vi "initial_feedback.vi"(1 "input cluster":T3) -> (0 "output cluster":T4)   [LabVIEW 2015]
uses:
  <vilib>/vision/Avi1.llb/AviRefnum.ctl
  <vilib>/userdefined/High Color/IMAQdx.ctl
  MWT.dll
panel:
  out "return type 2":i32
  out "return type":i32
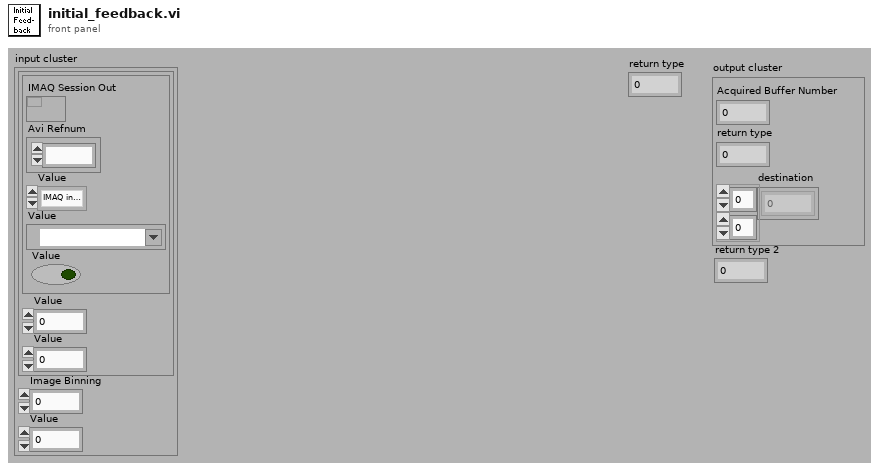
[diagram p1: front panel]
types:
  T1 = typedef "AviRefnum.ctl" = refnum<k1>
  T2 = typedef "IMAQdx.ctl" = refnum<k21>
  T3 = cluster{cluster{cluster{"IMAQ Session Out":refnum<k11>, "Avi Refnum":T1, "Value":enum32{"IMAQ interface", "IMAQdx interface", "AVI file"}, "Value":T2, "Value":bool}, "Value":i32, "Value":i32}, "Image Binning":u16, "Value":u16}
  T4 = cluster{"Acquired Buffer Number":i32, "return type":i32, "destination":i16[][]}
  T5 = typedef "Image Type" = u32
  T6 = typedef "IMAQ Image.ctl" = refnum<image>
  T7 = cluster{cluster{"IMAQ Session Out":refnum<k11>, "Avi Refnum":T1, "Value":enum32{"IMAQ interface", "IMAQdx interface", "AVI file"}, "Value":T2, "Value":bool}, "Value":i32, "Value":i32}
  T8 = cluster{"IMAQ Session Out":refnum<k11>, "Avi Refnum":T1, "Value":enum32{"IMAQ interface", "IMAQdx interface", "AVI file"}, "Value":T2, "Value":bool}
  T9 = cluster{cluster{"IMAQ Session Out":refnum<k11>, "Avi Refnum":T1, "Value":enum32{"IMAQ interface", "IMAQdx interface", "AVI file"}, "Value":T2, "Value":bool}, "Value":i32}
  T10 = cluster{"Acquired Buffer Number":i32, "return type":i32, "image":i16[][]}
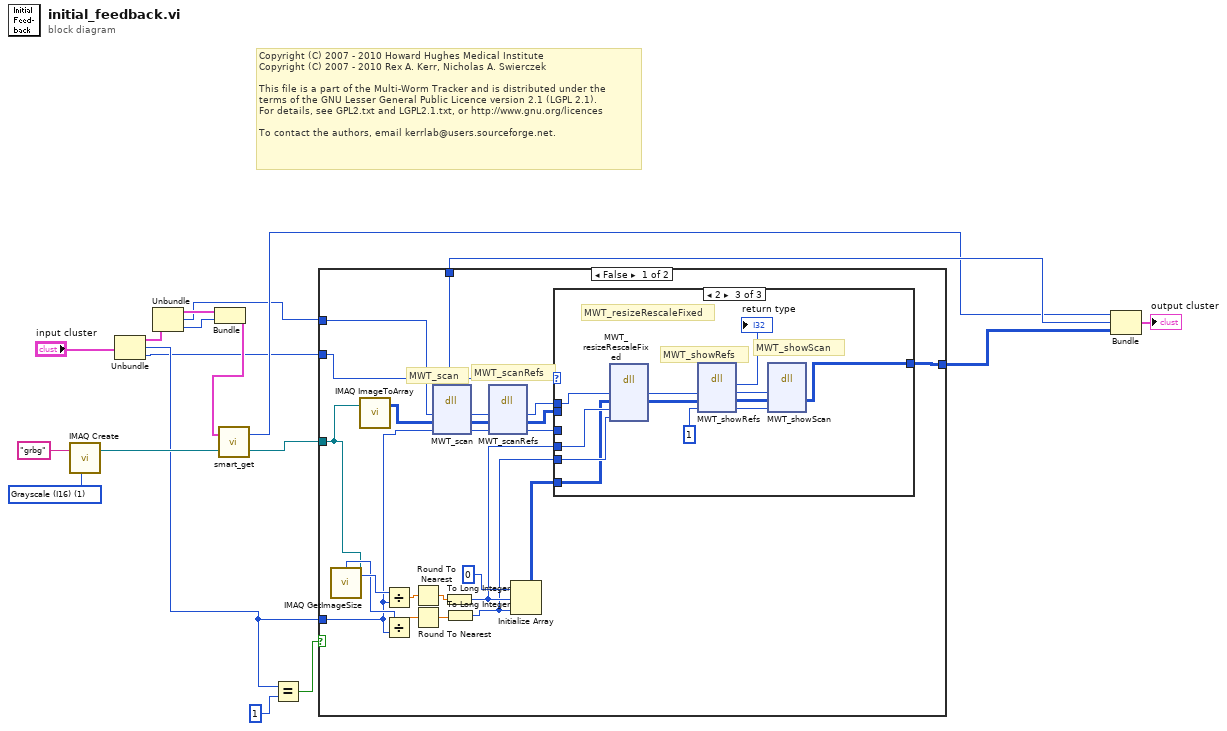
[diagram p0: block diagram]
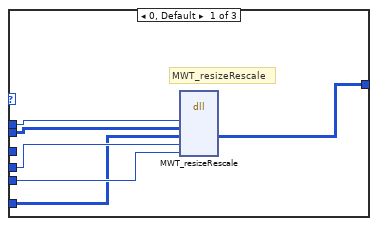
[diagram p2: hidden frame]
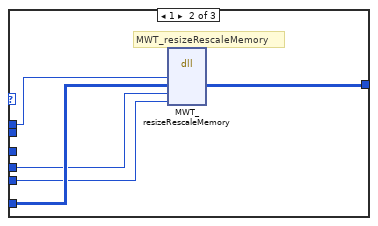
[diagram p3: hidden frame]
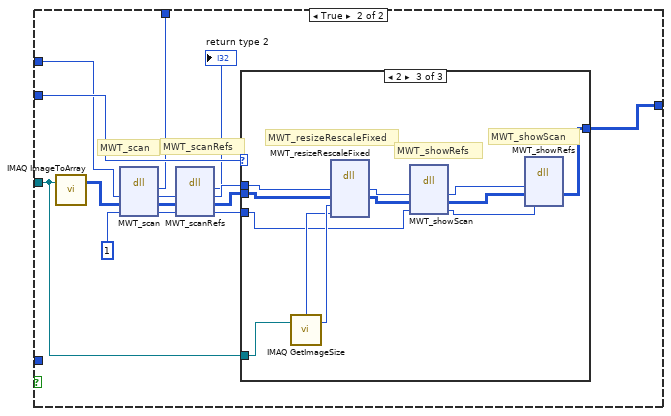
[diagram p4: hidden frame]
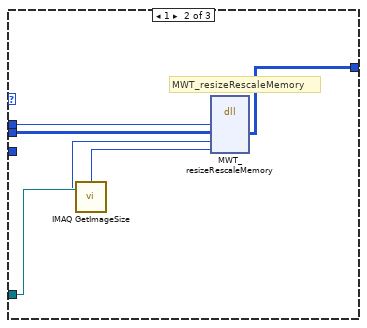
[diagram p6: hidden frame]
diagram:
  w16 = T5 1 items=["Grayscale (U8)", "Grayscale (I16)", "Grayscale (SGL)", "Complex (CSG)", "RGB (U32)", "HSL (U32)", "RGB (U64)"] ("Image Type")
  # "Copyright (C) 2007 - 2010 Howard Hughes Medical Institute\nCopyright (C) 2007 - 2010 Rex A. Kerr, Nicholas A. Swierczek\n \nThis file is a part of the Multi-Worm Tracker and is distributed under the\nterms of the GNU Lesser General Public Licence version 2.1 (LGPL 2.1).\nFor details, see GPL2.txt and LGPL2.1.txt, or http://www.gnu.org/licences\n \nTo contact the authors, email kerrlab@users.sourceforge.net."
  n1 = call "IMAQ Create"("Image Name"="grbg", "Image Type"=w16) -> ("New Image"=w13:T6)  [unwired: 3 in, 1 out]
  n2 = Unbundle("input cluster") -> (w8:T7, "Image Binning"=w9:u16, "Value"=w4:u16)
  n3 = Unbundle(w8) -> (w7:T8, "Value"=w3:i32, "Value"=w6:i32)
  n4 = Bundle(w7, "Value"=w6) -> (w5:T9)  [unwired: 1 in]
  n5 = call "smart_get.vi"("Input Image"=w13, "Cluster"=w5) -> ("Image Out"=w14:T6, "Acquired Buffer Number"=w10:i32)
  n6 = Equal?(x=w9, y=1) -> (x = y?=w17:bool)
  n7 = case shown="False" w17 {
    tunnel: w14 -> [w24 w65]
    tunnel: [w29 w67] -> w11
    tunnel: w4 -> [w30 w73]
    tunnel: [w28 w72] -> w12
    tunnel: w9 -> [w21 _]
    tunnel: w3 -> [w22 w71]
    frame False {
      # "MWT_scanRefs"
      # "MWT_scan"
      n8 = call "IMAQ GetImageSize"("Image"=w24) -> ("Y Resolution"=w41:i32, "X Resolution"=w40:i32)  [unwired: 3 in, 1 out]
      n9 = call "IMAQ ImageToArray"("Image"=w24) -> ("Image Pixels (I16)"=w23:i16[][])  [unwired: 3 in, 4 out]
      n10 = Divide(x=w41, y=w21) -> (x/y=w38:dbl)
      n11 = Divide(x=w40, y=w21) -> (x/y=w37:dbl)
      n12 = Round To Nearest(number=w38) -> (nearest integer value=w36:dbl)
      n13 = Round To Nearest(number=w37) -> (nearest integer value=w35:dbl)
      n14 = dll-call lib="C:/Users/ramasamyl/Desktop/MWT/MWT.dll" fn="MWT_scan"("handle"=w22, "image"=w23, "bin"=w21) -> ("return type"=w29:i32, "handle"=w32:i32, "image"=w31:i16[][], "bin"=w20:i32)  [unwired: 3 in, 2 out]
      n15 = To Long Integer(number=w36) -> (32bit integer=w26:i32)
      n16 = To Long Integer(number=w35) -> (32bit integer=w25:i32)
      n17 = dll-call lib="C:/Users/ramasamyl/Desktop/MWT/MWT.dll" fn="MWT_scanRefs"("handle"=w32, "image"=w31, "bin"=w20) -> ("handle"=w34:i32, "image"=w33:i16[][], "bin"=w19:i32)  [unwired: 4 in, 2 out]
      n18 = Initialize Array(i16 0 ("element"), w26, w25) -> (w27:i16[][])
      n19 = case shown="2" w30 {
        tunnel: w33 -> [w46 _ _]
        tunnel: w34 -> [w47 w51 w59]
        tunnel: [w42 w52 w53] -> w28
        tunnel: w27 -> [w43 w50 w55]
        tunnel: w26 -> [w45 w49 w57]
        tunnel: w25 -> [w44 w48 w56]
        tunnel: w19 -> [_ _ _]
        frame 0, Default {
          # "MWT_resizeRescale"
          n20 = dll-call lib="C:/Users/ramasamyl/Desktop/MWT/MWT.dll" fn="MWT_resizeRescale"("handle"=w47, "source"=w46, "destination"=w43, "width"=w45, "height"=w44) -> ("destination"=w42:i16[][])  [unwired: 8 in, 2 out]
        }
        frame 1 {
          # "MWT_resizeRescaleMemory"
          n21 = dll-call lib="C:/Users/ramasamyl/Desktop/MWT/MWT.dll" fn="MWT_resizeRescaleMemory"("handle"=w51, "destination"=w50, "width"=w49, "height"=w48) -> ("destination"=w52:i16[][])  [unwired: 7 in, 2 out]
        }
        frame 2 {
          # "MWT_resizeRescaleFixed"
          # "MWT_showScan"
          # "MWT_showRefs"
          n22 = dll-call lib="C:/Users/ramasamyl/Desktop/MWT/MWT.dll" fn="MWT_resizeRescaleFixed"("handle"=w59, "destination"=w55, "width"=w57, "height"=w56) -> ("handle"=w58:i32, "destination"=w54:i16[][])  [unwired: 6 in, 2 out]
          n23 = dll-call lib="C:/Users/ramasamyl/Desktop/MWT/MWT.dll" fn="MWT_showRefs"("handle"=w58, "image"=w54, "binning"=1) -> ("return type"=→"return type":i32, "handle"=w64:i32, "image"=w63:i16[][], "binning"=w62:i32)  [unwired: 3 in, 2 out]
          n24 = dll-call lib="C:/Users/ramasamyl/Desktop/MWT/MWT.dll" fn="MWT_showScan"("handle"=w64, "image"=w63, "binning"=w62) -> ("image"=w53:i16[][])  [unwired: 6 in, 2 out]
        }
      }
    }
    frame True {
      # "MWT_scanRefs"
      # "MWT_scan"
      n25 = call "IMAQ ImageToArray"("Image"=w65) -> ("Image Pixels (I16)"=w74:i16[][])  [unwired: 3 in, 4 out]
      n26 = dll-call lib="C:/Users/ramasamyl/Desktop/MWT/MWT.dll" fn="MWT_scan"("handle"=w71, "image"=w74, "bin"=1) -> ("return type"=w67:i32, "handle"=w76:i32, "image"=w75:i16[][], "bin"=w69:i32)  [unwired: 3 in, 2 out]
      n27 = dll-call lib="C:/Users/ramasamyl/Desktop/MWT/MWT.dll" fn="MWT_scanRefs"("handle"=w76, "image"=w75, "bin"=w69) -> ("return type"=→"return type 2":i32, "handle"=w78:i32, "image"=w77:i16[][], "bin"=w68:i32)  [unwired: 3 in, 2 out]
      n28 = case shown="2" w73 {
        tunnel: w77 -> [w79 w80 w87]
        tunnel: w78 -> [_ w81 w86]
        tunnel: [w79 w82 w94] -> w72
        tunnel: w65 -> [_ w85 w97]
        tunnel: w68 -> [_ _ w91]
        frame 0, Default {
        }
        frame 1 {
          # "MWT_resizeRescaleMemory"
          n29 = call "IMAQ GetImageSize"("Image"=w85) -> ("Y Resolution"=w84:i32, "X Resolution"=w83:i32)  [unwired: 3 in, 1 out]
          n30 = dll-call lib="C:/Users/ramasamyl/Desktop/MWT/MWT.dll" fn="MWT_resizeRescaleMemory"("handle"=w81, "destination"=w80, "width"=w84, "height"=w83) -> ("destination"=w82:i16[][])  [unwired: 7 in, 2 out]
        }
        frame 2 {
          # "MWT_showScan"
          # "MWT_resizeRescaleFixed"
          # "MWT_showRefs"
          n31 = call "IMAQ GetImageSize"("Image"=w97) -> ("Y Resolution"=w96:i32, "X Resolution"=w95:i32)  [unwired: 3 in, 1 out]
          n32 = dll-call lib="C:/Users/ramasamyl/Desktop/MWT/MWT.dll" fn="MWT_resizeRescaleFixed"("handle"=w86, "destination"=w87, "width"=w96, "height"=w95) -> ("handle"=w93:i32, "destination"=w92:i16[][])  [unwired: 6 in, 2 out]
          n33 = dll-call lib="C:/Users/ramasamyl/Desktop/MWT/MWT.dll" fn="MWT_showScan"("handle"=w93, "image"=w92, "bin"=w91) -> ("handle"=w89:i32, "image"=w88:i16[][], "bin"=w90:i32)  [unwired: 4 in, 2 out]
          n34 = dll-call lib="C:/Users/ramasamyl/Desktop/MWT/MWT.dll" fn="MWT_showRefs"("handle"=w89, "image"=w88, "bin"=w90) -> ("image"=w94:i16[][])  [unwired: 6 in, 2 out]
        }
      }
    }
  }
  n35 = Bundle("Acquired Buffer Number"=w10, "return type"=w11, "image"=w12) -> (→"output cluster":T10)  [unwired: 1 in]
